vi "Get Linker Errors.vi"(8 "error in (no error)":errorcluster, 11 "NI_AB_API_Build in":refnum<class "NI_AB_API_Build.lvclass">) -> (0 "error out":errorcluster, 2 "Missing VIs Call Chain":variant, 3 "NI_AB_API_Build out":refnum<class "NI_AB_API_Build.lvclass">, 5 "Has errors?":bool=TRUE)   [LabVIEW 2020, in "NI_AB_API_Build.lvclass"]
uses:
  <vilib>/AppBuilder/AB_API/Build/NI_AB_API_Build.lvclass
  <vilib>/AppBuilder/AB_API/Build/NI_AB_API_Build.lvclass/NI_AB_API_Build.ctl
  <vilib>/AppBuilder/AB_Classes/Build/AB_Build.lvclass
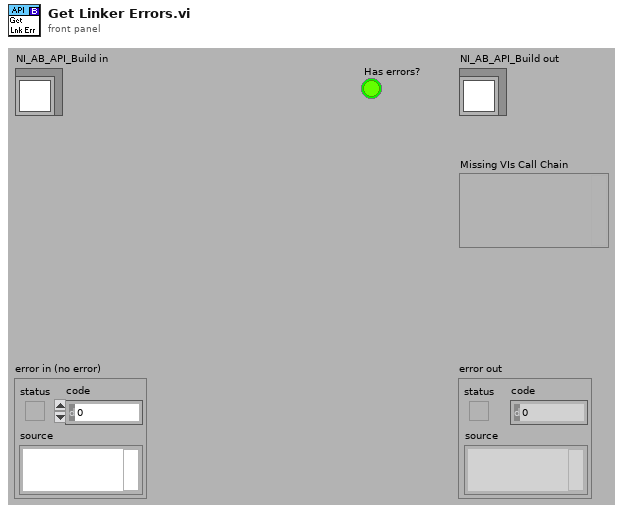
[diagram p1: front panel]
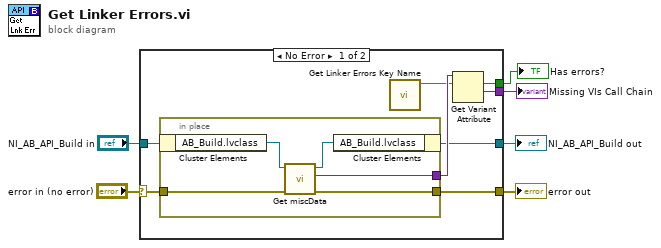
[diagram p0: block diagram]
diagram:
  n1 = case shown="No Error" "error in (no error)" {
    selector: "error in (no error)" -> [w14 w21]
    tunnel: [w13 w21] -> w5
    tunnel: [w8 w20] -> w3
    tunnel: "NI_AB_API_Build in" -> [w9 w20]
    tunnel: [w12 _] -> w2
    tunnel: [w11 _] -> w1
    frame No Error {
      n2 = in-place {
        in-place-border: w14 -> [w19]
        in-place-border: [w18] -> w13
        in-place-border: [w17] -> w10
        n3 = in-place-cluster #1(w9) -> ("AB_Build.lvclass"=w16:refnum<class "AB_Build.lvclass">)
        n4 = call-dynamic "Get miscData.vi"("error in (no error)"=w19, "AB_Build in"=w16) -> ("error out"=w18:errorcluster, "eng_miscData"=w17:variant, "AB_Build out"=w15:refnum<class "AB_Build.lvclass">)  [unwired: 7 in]
        n5 = in-place-cluster #1("AB_Build.lvclass"=w15) -> (w8:refnum<class "NI_AB_API_Build.lvclass">)
      }
      n6 = call <vilib>:"Get Linker Errors Key Name.vi"() -> ("broken vis errors key"=w7:string)  [unwired: 10 in, 1 out]
      n7 = Get Variant Attribute(Variant=w10, name=w7) -> (found=w11:bool, value=w12:variant)  [unwired: 2 in, 2 out]
    }
    frame Error {
    }
  }
  "error out" <- w5
  "NI_AB_API_Build out" <- w3
  "Missing VIs Call Chain" <- w2
  "Has errors?" <- w1
